vi "Serial Port Instructions.vi"() -> ()   [LabVIEW 2013]
uses:
  <vilib>/Instr/_visa.llb/VISA Configure Serial Port (Instr).vi
panel:
  in  "parameter":u8
  in  "command":u8
  in  "Serial port":refnum<visa-resource-name>
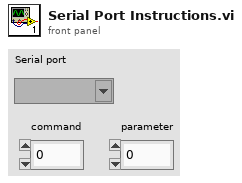
[diagram p1: front panel]
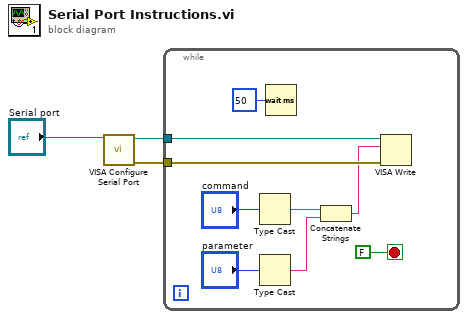
[diagram p0: block diagram]
diagram:
  n1 = call-poly "VISA Configure Serial Port"("VISA resource name"="Serial port") -> ("VISA resource name out"=w2:refnum<visa-resource-name>, "error out"=w1:errorcluster)  [unwired: 13 in]
  n2 = while {
    tunnel: w2 -> [w12]
    tunnel: w1 -> [w11]
    stop <- FALSE stop-if-true
    n3 = Type Cast(x="command") -> (*(type *) &x=w6:string)  [unwired: 1 in]
    n4 = Type Cast(x="parameter") -> (*(type *) &x=w5:string)  [unwired: 1 in]
    n5 = Wait (ms)(milliseconds to wait=u32 50) -> ()  [unwired: 1 out]
    n6 = Concatenate Strings(w6, w5) -> (w4:string)
    n7 = VISA Write(VISA resource name=w12, write buffer=w4, error in (no error)=w11) -> ()  [unwired: 3 out]
  }
